vi "DIO Write.vi"(1 "Data":bool[](array[boolean]), 2 "Channels":i32[](array[numeric]), 3 "device":i16=1) -> (0 "Error":bool)   [LabVIEW 2009]
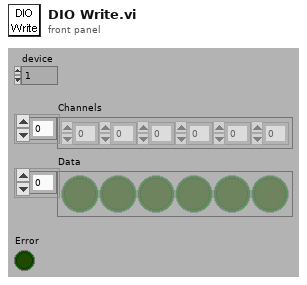
[diagram p1: front panel]
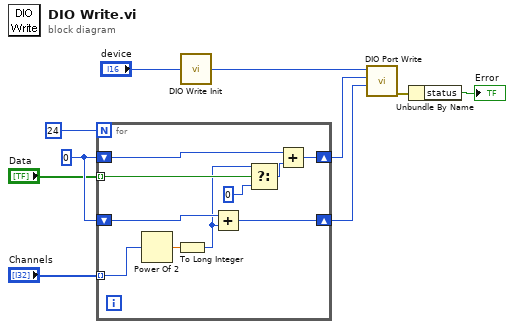
[diagram p0: block diagram]
diagram:
  w8 = 0
  n1 = for {
    N: i16 24 ("port width") -> [_]
    tunnel: "Channels" -> [w12] mode=indexing
    shift-right: [w19] -> w5
    shift-left: w8 -> [w18]
    shift-right: [w16] -> w6
    shift-left: w8 -> [w14]
    tunnel: "Data" -> [w13] mode=indexing
    n2 = Power Of 2(x=w12) -> (2^x=w20:dbl)
    n3 = To Long Integer(number=w20) -> (32bit integer=w11:i32)
    n4 = Add(x=w18, y=w11) -> (x+y=w19:i32)
    n5 = Select(t=w11, s=w13, f=0) -> (s? t:f=w15:i32)
    n6 = Add(x=w14, y=w15) -> (x+y=w16:i32)
  }
  n7 = call "DIO Write Init.vi"("device"="device") -> ("task ID out"=w10:u32)
  n8 = call <vilib>:"DIO Port Write.vi"("line mask"=w5, "pattern"=w6, "task ID"=w10) -> ("error out"=w1:errorcluster)  [unwired: 7 in, 1 out]
  n9 = Unbundle By Name(w1) -> ("status"=→"Error":bool)
